vi "IsCorrect.vi"(0 "Boolean":bool, 1 "InValue":i32, 5 "Boolean 2":bool, 9 "Boolean 3":bool, 11 "Boolean 4":bool) -> (4 "IsCorrect":bool)   [LabVIEW 2025]
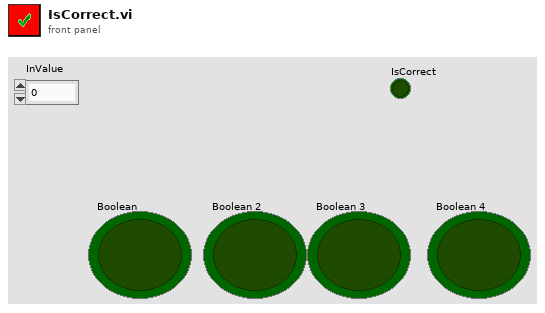
[diagram p1: front panel]
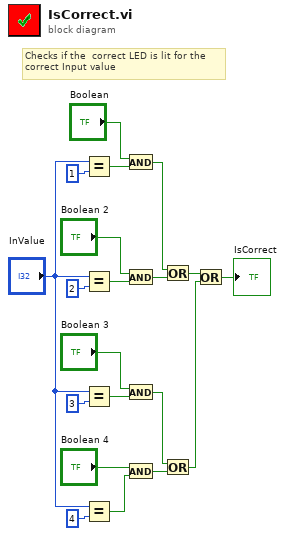
[diagram p0: block diagram]
diagram:
  # "Checks if the  correct LED is lit for the \ncorrect Input value"
  n1 = Equal?(x="InValue", y=1) -> (x = y?=w8:bool)
  n2 = Equal?(x="InValue", y=2) -> (x = y?=w2:bool)
  n3 = Equal?(x="InValue", y=3) -> (x = y?=w4:bool)
  n4 = Equal?(x="InValue", y=4) -> (x = y?=w6:bool)
  n5 = And(x="Boolean", y=w8) -> (x .and. y?=w16:bool)
  n6 = And(x="Boolean 2", y=w2) -> (x .and. y?=w15:bool)
  n7 = And(x="Boolean 3", y=w4) -> (x .and. y?=w14:bool)
  n8 = And(x="Boolean 4", y=w6) -> (x .and. y?=w13:bool)
  n9 = Or(x=w16, y=w15) -> (x .or. y?=w12:bool)
  n10 = Or(x=w14, y=w13) -> (x .or. y?=w11:bool)
  n11 = Or(x=w12, y=w11) -> (x .or. y?=→"IsCorrect":bool)
